vi "LCDStart.vi"(0 "Device Info":T1={"Serial Number"=-1, "Channel"=0, "Port"=0}, 1 "Contrast":dbl=0.25, 2 "Backlight":dbl, 3 "Screen Size":u32(ring)=7 items=["SCREEN_SIZE_NONE"=1, "SCREEN_SIZE_1x8"=2, "SCREEN_SIZE_2x8"=3, "SCREEN_SIZE_1x16"=4, "SCREEN_SIZE_2x16"=5, "SCREEN_SIZE_4x16"=6, "SCREEN_SIZE_2x20"=7, "SCREEN_SIZE_4x20"=8, "SCREEN_SIZE_2x24"=9, "SCREEN_SIZE_1x40"=10, "SCREEN_SIZE_2x40"=11, "SCREEN_SIZE_4x40"=12, "SCREEN_SIZE_64x128"=13], 11 "error in (no error)":errorcluster, 12 "Connection":u16(ring) items=["No Preference", "Remote", "Local"], 13 "Timeout (mSec)":i32=5000) -> (4 "Phidget ID":u64, 6 "Serial Number Return":i32, 10 "Attached?":bool, 15 "error out":errorcluster)   [LabVIEW 2012, in "Phidget LCD.lvlib"]
doc: "${LCD:StartHeader}"
uses:
  <instrlib>/Phidgets/Phidget LCD/Phidget LCD.lvlib
  <instrlib>/Phidgets/Phidget Common/Phidget Common.lvlib
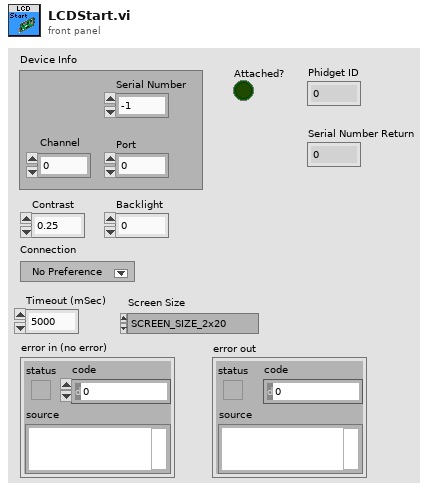
[diagram p1: front panel]
types:
  T1 = cluster{"Serial Number":i32, "Channel":i32, "Port":i32}
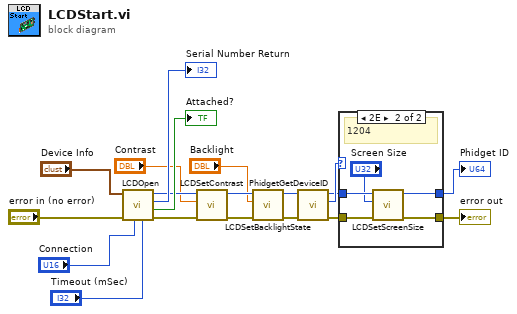
[diagram p0: block diagram]
diagram:
  n1 = call <instrlib>:"LCDOpen.vi"("Timeout (mSec)"="Timeout (mSec)", "Connection"="Connection", "error in"="error in (no error)", "Device Info"="Device Info") -> ("error out"=w11:errorcluster, "Attached?"=→"Attached?":bool, "Serial Number Return"=→"Serial Number Return":i32, "Phidget ID"=w12:u64)  [unwired: 4 in]
  n2 = call <instrlib>:"LCDSetContrast.vi"("error in (no error)"=w11, "Contrast"="Contrast", "Device In"=w12) -> ("error out"=w14:errorcluster, "Device Out"=w13:u64)  [unwired: 6 in]
  n3 = call <instrlib>:"LCDSetBacklightState.vi"("error in (no error)"=w14, "Backlight"="Backlight", "Device In"=w13) -> ("error out"=w7:errorcluster, "Device Out"=w6:u64)  [unwired: 6 in]
  n4 = call <instrlib>:"PhidgetGetDeviceID.vi"("error in (no error)"=w7, "Device In"=w6) -> ("error out"=w3:errorcluster, "Devie IDs"=w5:u32, "Device Out"=w4:u64)  [unwired: 6 in]
  n5 = case shown="2E" w5 {
    tunnel: w4 -> [w21 w25]
    tunnel: w3 -> [w20 w26]
    tunnel: [w21 w24] -> w2
    tunnel: [w20 w23] -> w1
    frame 0, Default {
    }
    frame 46 {
      # "1204"
      n6 = call <instrlib>:"LCDSetScreenSize.vi"("error in (no error)"=w26, "Screen Size"="Screen Size", "Device In"=w25) -> ("error out"=w23:errorcluster, "Device Out"=w24:u64)  [unwired: 6 in]
    }
  }
  "error out" <- w1
  "Phidget ID" <- w2
